vi "GlobalSettings.Create.vi"(8 "error in (no error)":errorcluster, 11 "Device Item Ref in":T1 format="%.0x") -> (0 "error out":errorcluster, 3 "Parent Ref out":T1 format="%.0x")   [LabVIEW 2015, in "Fuel Injector Analysis Addon System Explorer.lvlib"]
uses:
  Fuel Injector Analysis Addon System Explorer.lvlib
  <vilib>/NI Veristand/Custom Device API/Custom Device Item Ref.ctl
  <vilib>/NI Veristand/Custom Device API/Custom Device Channel.ctl
  <vilib>/NI Veristand/Custom Device API/Custom Device Channel Type.ctl
  Shared/Constants.vi
  <vilib>/NI Veristand/Custom Device API/Custom Device API.lvlib
  Shared/Fuel Injector Analysis Addon Shared.lvlib
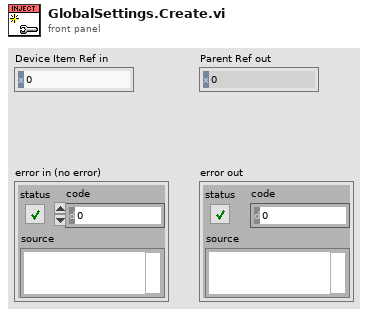
[diagram p1: front panel]
types:
  T1 = typedef "Custom Device API.lvlib/Custom Device Item Ref.ctl" = u64
  T2 = typedef "Custom Device API.lvlib/Custom Device Channel.ctl" = cluster{"Type":T3, "Units":string, "Default Value":dbl, "Faultable":bool, "Scalable":bool}
  T3 = typedef "Custom Device API.lvlib/Custom Device Channel Type.ctl" = enum16{"Input", "Output"}
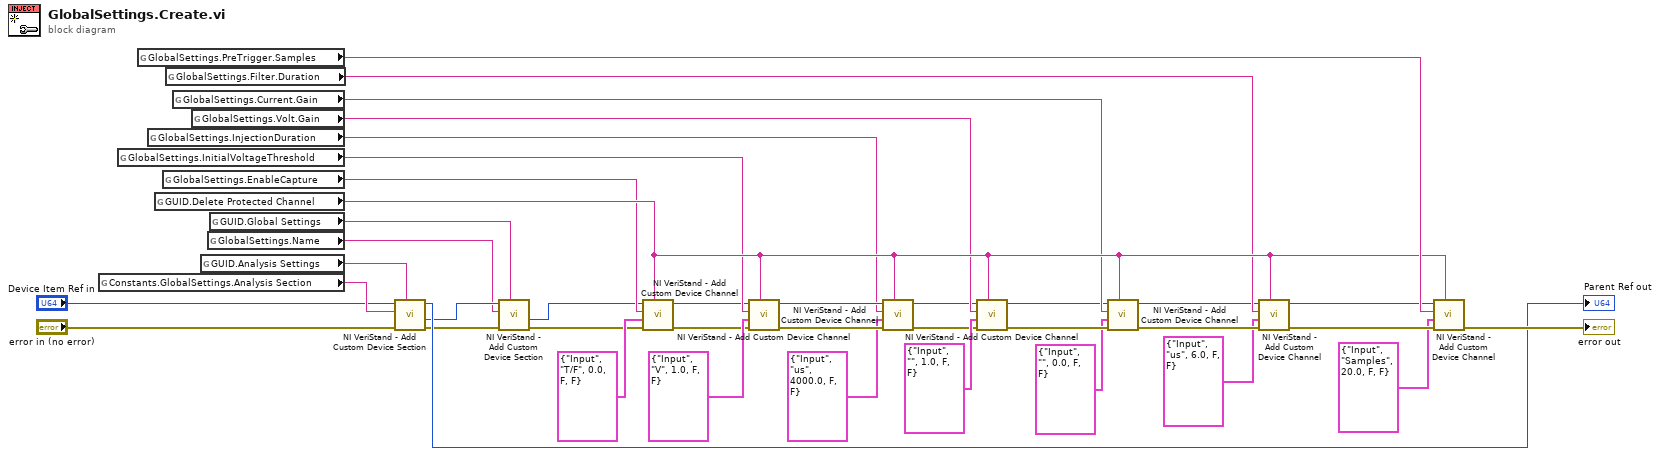
[diagram p0: block diagram]
diagram:
  n1 = global read "Constants.vi" "Constants.GlobalSettings.Analysis Section"() -> (w20:string)
  n2 = global read "Constants.vi" "GlobalSettings.InitialVoltageThreshold"() -> (w27:string)
  n3 = global read "Constants.vi" "GlobalSettings.PreTrigger.Samples"() -> (w39:string)
  n4 = global read "Constants.vi" "GlobalSettings.InjectionDuration"() -> (w14:string)
  n5 = global read "Constants.vi" "GUID.Delete Protected Channel"() -> (w38:string)
  n6 = global read "Constants.vi" "GlobalSettings.EnableCapture"() -> (w13:string)
  n7 = global read "Constants.vi" "GlobalSettings.Filter.Duration"() -> (w37:string)
  n8 = global read "Constants.vi" "GlobalSettings.Current.Gain"() -> (w16:string)
  n9 = global read "Constants.vi" "GlobalSettings.Volt.Gain"() -> (w15:string)
  n10 = global read "Constants.vi" "GUID.Analysis Settings"() -> (w21:string)
  n11 = global read "Constants.vi" "GlobalSettings.Name"() -> (w4:string)
  n12 = global read "Constants.vi" "GUID.Global Settings"() -> (w1:string)
  n13 = call <vilib>:"NI VeriStand - Add Custom Device Section.vi"("GUID (Default Section)"=w21, "error in (no error)"="error in (no error)", "Section Name"=w20, "Parent Ref in"="Device Item Ref in") -> ("error out"=w18:errorcluster, "Section Ptr"=w22:T1, "Parent Ref out"=→"Parent Ref out":T1)  [unwired: 4 in, 1 out]
  n14 = call <vilib>:"NI VeriStand - Add Custom Device Section.vi"("GUID (Default Section)"=w1, "error in (no error)"=w18, "Section Name"=w4, "Parent Ref in"=w22) -> ("error out"=w2:errorcluster, "Section Ptr"=w3:T1)  [unwired: 4 in, 2 out]
  n15 = call <vilib>:"NI VeriStand - Add Custom Device Channel.vi"("GUID (Default Channel)"=w38, "error in (no error)"=w2, "Channel"=T2 {"Type"=enum."Input", "Units"="T/F", "Default Value"=0.0, "Faultable"=FALSE, "Scalable"=FALSE}, "Channel Name"=w13, "Parent Ref in"=w3) -> ("error out"=w24:errorcluster, "Parent Ref out"=w25:T1)  [unwired: 3 in, 2 out]
  n16 = call <vilib>:"NI VeriStand - Add Custom Device Channel.vi"("GUID (Default Channel)"=w38, "error in (no error)"=w24, "Channel"=T2 {"Type"=enum."Input", "Units"="V", "Default Value"=1.0, "Faultable"=FALSE, "Scalable"=FALSE}, "Channel Name"=w27, "Parent Ref in"=w25) -> ("error out"=w28:errorcluster, "Parent Ref out"=w29:T1)  [unwired: 3 in, 2 out]
  n17 = call <vilib>:"NI VeriStand - Add Custom Device Channel.vi"("GUID (Default Channel)"=w38, "error in (no error)"=w28, "Channel"=T2 {"Type"=enum."Input", "Units"="us", "Default Value"=4000.0, "Faultable"=FALSE, "Scalable"=FALSE}, "Channel Name"=w14, "Parent Ref in"=w29) -> ("error out"=w8:errorcluster, "Parent Ref out"=w7:T1)  [unwired: 3 in, 2 out]
  n18 = call <vilib>:"NI VeriStand - Add Custom Device Channel.vi"("GUID (Default Channel)"=w38, "error in (no error)"=w8, "Channel"=T2 {"Type"=enum."Input", "Units"="", "Default Value"=1.0, "Faultable"=FALSE, "Scalable"=FALSE}, "Channel Name"=w15, "Parent Ref in"=w7) -> ("error out"=w12:errorcluster, "Parent Ref out"=w11:T1)  [unwired: 3 in, 2 out]
  n19 = call <vilib>:"NI VeriStand - Add Custom Device Channel.vi"("GUID (Default Channel)"=w38, "error in (no error)"=w12, "Channel"=T2 {"Type"=enum."Input", "Units"="", "Default Value"=0.0, "Faultable"=FALSE, "Scalable"=FALSE}, "Channel Name"=w16, "Parent Ref in"=w11) -> ("error out"=w32:errorcluster, "Parent Ref out"=w33:T1)  [unwired: 3 in, 2 out]
  n20 = call <vilib>:"NI VeriStand - Add Custom Device Channel.vi"("GUID (Default Channel)"=w38, "error in (no error)"=w32, "Channel"=T2 {"Type"=enum."Input", "Units"="us", "Default Value"=6.0, "Faultable"=FALSE, "Scalable"=FALSE}, "Channel Name"=w37, "Parent Ref in"=w33) -> ("error out"=w34:errorcluster, "Parent Ref out"=w35:T1)  [unwired: 3 in, 2 out]
  n21 = call <vilib>:"NI VeriStand - Add Custom Device Channel.vi"("GUID (Default Channel)"=w38, "error in (no error)"=w34, "Channel"=T2 {"Type"=enum."Input", "Units"="Samples", "Default Value"=20.0, "Faultable"=FALSE, "Scalable"=FALSE}, "Channel Name"=w39, "Parent Ref in"=w35) -> ("error out"=→"error out":errorcluster)  [unwired: 3 in, 3 out]
